vi "Read Data.vi"(8 "error in (no error)":errorcluster, 11 "Send Data to Caller in":refnum<class "Send Data to Caller.lvclass">) -> (0 "error out":errorcluster, 2 "Base Data Lib:Data":refnum<class "Data.lvclass">, 3 "Send Data to Caller out":refnum<class "Send Data to Caller.lvclass">)   [LabVIEW 2014, in "Send Data to Caller.lvclass"]
uses:
  Send Data to Caller.lvclass
  Data/Data.lvclass
  Send Data to Caller.lvclass/Send Data to Caller.ctl
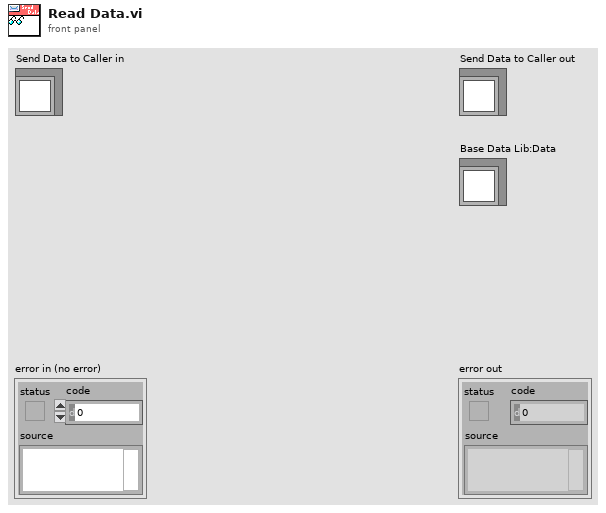
[diagram p1: front panel]
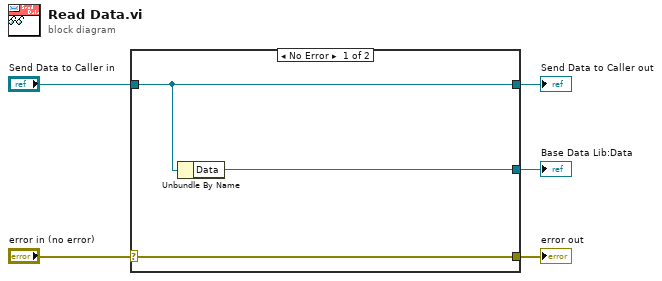
[diagram p0: block diagram]
diagram:
  n1 = case shown="No Error" "error in (no error)" {
    selector: "error in (no error)" -> [w8 w9]
    tunnel: [w8 w9] -> w4
    tunnel: [w7 w10] -> w2
    tunnel: "Send Data to Caller in" -> [w7 w10]
    tunnel: [w6 _] -> w1
    frame No Error {
      n2 = Unbundle By Name(w7) -> ("Data"=w6:refnum<class "Data.lvclass">)
    }
    frame Error {
    }
  }
  "error out" <- w4
  "Send Data to Caller out" <- w2
  "Base Data Lib:Data" <- w1
